vi "Save.vi"(8 "error in (no error)":errorcluster, 9 "File Path":path, 10 "TDMS File Writer in":refnum<class "File Writer_TDMS.lvclass">, 11 "Data":refnum<class "Data.lvclass">) -> (0 "error out":errorcluster, 2 "Actor out":refnum<class "Actor.lvclass">)   [LabVIEW 2020, in "File Writer_TDMS.lvlib" / "File Writer_TDMS.lvclass"]
doc: "Save 'Data' to the active TDMS file."
uses:
  File Writer_TDMS.lvclass
  C:/Current projects/WS/PPL/HDH.Actor Framework.Core.Actor.lvlibp/1abvi3w/vi.lib/ActorFramework/Actor/Actor.lvclass
  PPL/HDH.Actor Framework.Core.Actor.lvlibp/1abvi3w/vi.lib/ActorFramework/Actor/Actor.lvclass
  PPL/HDH.Data.Generic.lvlibp/Data.lvclass
  File Writer_TDMS.lvclass/File Writer_TDMS.ctl
  PPL/HDH.Data.Generic.FileIO.TDMS.lvlibp
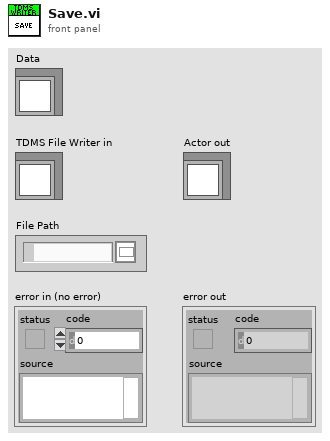
[diagram p1: front panel]
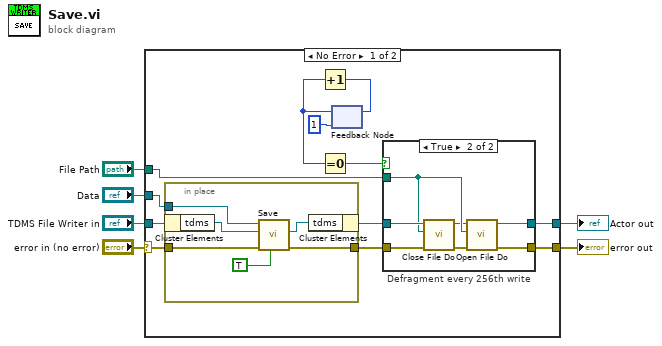
[diagram p0: block diagram]
diagram:
  n1 = case shown="No Error" "error in (no error)" {
    selector: "error in (no error)" -> [w16 w34]
    tunnel: "TDMS File Writer in" -> [w18 w35]
    tunnel: "Data" -> [w17 _]
    tunnel: [w10 w35] -> w3
    tunnel: [w8 w34] -> w2
    tunnel: "File Path" -> [w7 _]
    frame No Error {
      n2 = in-place {
        in-place-border: w17 -> [w33]
        in-place-border: w16 -> [w31]
        in-place-border: [w28] -> w11
        n3 = in-place-cluster #1(w18) -> ("tdms"=w32:refnum<k34>)
        n4 = call "Save.vi"("Force Single Line(T)"=TRUE, "error in (no error)"=w31, "TDMS in"=w32, "Data to Save"=w33) -> ("error out"=w28:errorcluster, "TDMS Out"=w29:refnum<k34>)  [unwired: 6 in]
        n5 = in-place-cluster #1("tdms"=w29) -> (w9:refnum<class "File Writer_TDMS.lvclass">)
      }
      n6 = feedback #2(u8 1) -> (w14:u8)
      n7 = Increment(x=w14) -> (x+1=w13:u8)
      n8 = Equal To 0?(x=w14) -> (x = 0?=w15:bool)
      n9 = feedback-in #2(w13) -> ()
      n10 = case "Defragment every 256th write" shown="True" w15 {
        tunnel: w11 -> [w19 w26]
        tunnel: [w20 w23] -> w10
        tunnel: w9 -> [w20 w27]
        tunnel: [w19 w21] -> w8
        tunnel: w7 -> [_ w25]
        frame False {
        }
        frame True {
          n11 = call-dynamic "Close File Do.vi"("error in (no error)"=w26, "File Path"=w25, "TDMS File Writer in"=w27) -> ("error out"=w22:errorcluster, "TDMS File Writer out"=w24:refnum<class "File Writer_TDMS.lvclass">)  [unwired: 7 in]
          n12 = call-dynamic "Open File Do.vi"("error in (no error)"=w22, "New File Path"=w25, "TDMS File Writer in"=w24) -> ("error out"=w21:errorcluster, "TDMS File Writer out"=w23:refnum<class "File Writer_TDMS.lvclass">)  [unwired: 6 in, 1 out]
        }
      }
    }
    frame Error {
    }
  }
  "error out" <- w2
  "Actor out" <- w3
